vi "Get Project Types.vi"(10 "Project:Active Project":refnum<vi>) -> (2 "Type Name Library File Path":map{string, map{string, path}}(c390))   [LabVIEW 2020, in "_Shared.lvlib"]
uses:
  _Shared.lvlib
  jettl/jettl/Msg/Msg.lvclass
  jettl/jettl/Actor/Actor/Actor.lvclass
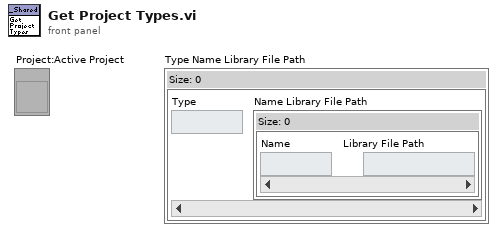
[diagram p1: front panel]
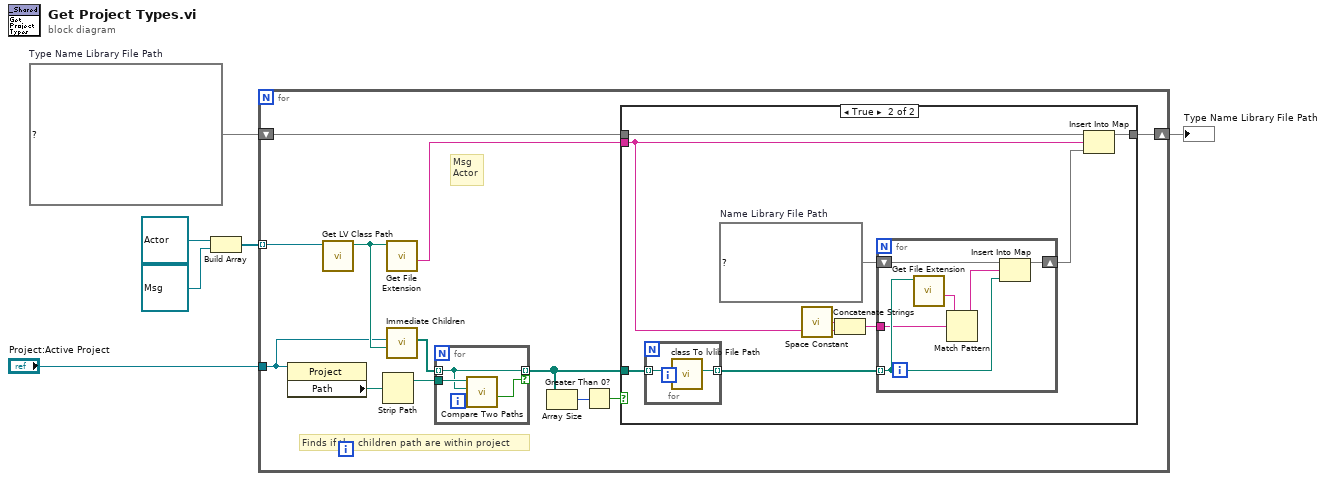
[diagram p0: block diagram]
diagram:
  w6 = map{string, map{string, path}} {}  # Type Name Library File Path
  n1 = Build Array(refnum<class "Actor.lvclass"> refnum ("jettl.lvlib:Actor.lvlib:Actor.lvclass"), refnum<class "Msg.lvclass"> refnum ("jettl.lvlib:Msg.lvclass")) -> (w5:refnum<class>[])
  n2 = for {
    shift-right: [w13] -> w3
    shift-left: w6 -> [w14]
    tunnel: w5 -> [w12] mode=indexing
    tunnel: "Project:Active Project" -> [w7]
    # "Msg\nActor"
    # "Finds if the children path are within project"
    n3 = property class="Project"(reference=w7) -> ("Path"=w10:path)  [unwired: 1 in, 2 out]
    n4 = call <vilib>:"Get LV Class Path.vi"("object"=w12) -> ("class path"=w8:path)  [unwired: 9 in, 1 out]
    n5 = Strip Path(path=w10) -> (stripped path=w9:path)  [unwired: 1 out]
    n6 = call <vilib>:"Get File Extension.vi"("file"=w8) -> ("filename without extension"=w11:string)  [unwired: 6 in, 4 out]
    n7 = call "Immediate Children.vi"("Type File Path"=w8, "Project:Active Project"=w7) -> ("Implemented Class File Paths"=w18:path[])  [unwired: 8 in, 1 out]
    n8 = for {
      tunnel: w18 -> [w37] mode=indexing
      tunnel: [w37] -> w16 mode=indexing if=w39
      tunnel: w9 -> [w38]
      n9 = call <vilib>:"Compare Two Paths.vi"("Path 2"=w37, "Path 1"=w38) -> ("Path 2 Relative to Path 1?"=w39:bool)  [unwired: 6 in, 3 out]
    }
    n10 = Array Size(array=w16) -> (size(s)=w17:i32)
    n11 = Greater Than 0?(x=w17) -> (x > 0?=w15:bool)
    n12 = case shown="True" w15 {
      tunnel: w16 -> [_ w24]
      tunnel: w11 -> [_ w21]
      tunnel: w14 -> [w19 w28]
      tunnel: [w19 w27] -> w13
      frame False {
      }
      frame True {
        w25 = map{string, path} {}  # Name Library File Path
        n13 = for {
          tunnel: w24 -> [w30] mode=indexing
          tunnel: [w29] -> w23 mode=indexing
          n14 = call "class To lvlib File Path.vi"("class File Path"=w30) -> ("lvlib File Path"=w29:path)  [unwired: 10 in]
        }
        n15 = call <vilib>:"Space Constant.vi"() -> ("String"=w22:string)
        n16 = Concatenate Strings(w22, w21) -> (w20:string)
        n17 = for {
          tunnel: w23 -> [w33] mode=indexing
          tunnel: w20 -> [w31]
          shift-right: [w35] -> w26
          shift-left: w25 -> [w36]
          n18 = call <vilib>:"Get File Extension.vi"("file"=w33) -> ("filename without extension"=w32:string)  [unwired: 6 in, 4 out]
          n19 = Match Pattern(string=w32, regular expression=w31) -> (before substring=w34:string)  [unwired: 1 in, 3 out]
          n20 = Insert Into Map(map in=w36, key=w34, value=w33) -> (map out=w35:map{string, path})  [unwired: 2 out]
        }
        n21 = Insert Into Map(map in=w28, key=w21, value=w26) -> (map out=w27:map{string, map{string, path}})  [unwired: 2 out]
      }
    }
  }
  "Type Name Library File Path" <- w3
